vi "毕设原版.vi"() -> ()   [LabVIEW 2018]
uses:
  <vilib>/Utility/NIReport.llb/Report Type.ctl
  <vilib>/addons/control/pid/pid.llb/PID (DBL).vi
  <vilib>/Utility/NIReport.llb/Append Report Text (str wrap).vi
  <vilib>/express/express arith-compare/Formula/XNode/ExpressFormulaBlockNode.xnode
  <vilib>/Utility/NIReport.llb/NI_report.lvclass
  <vilib>/addons/control/pid/NI_PID_pid.lvlib
  <vilib>/Utility/NIReport.llb/NI_ReportGenerationCore.lvlib
  <vilib>/Utility/NIReport.llb/Excel/NI_Excel.lvclass
  <vilib>/Utility/NIReport.llb/Append Text Table to Report (wrap).vi
panel:
  out "波形图表":dbl(graph)
  out "过程变量和设定值 2":cluster{dbl, "SP：":dbl}(graph)
  in  "停止 3":bool
  out "实验要求":string="超    调    振    \n调    节    荡\n量    时    频\n不    间    率\n超    小    小\n过    于    于\n10   15    0.7\n%     s   rad/s"
  in  "密码修改":bool
  out "error out 6":errorcluster caption="error out"
  out "error out 5":errorcluster caption="error out"
  out "error out 4":errorcluster caption="error out"
  out "Values":string
  out "Command Text":string
  out "error out 2":errorcluster caption="错误输出"
  out "y":dbl[](array[numeric])
  out "time":dbl[](array[numeric])
  out "source":string
  out "Data":string[][](array[string])=[["10152949", "987654", "student"], ["10152950", "123456", "student"], ["10152951", "654321", "teacher"], ["10152952", "283411", "administrator"]]
  out "error out 3":errorcluster caption="error out"
  in  "report file path":path=path "F:/LabVIEW练习/毕设/实验成绩.xls"
  out "尝试次数":u32
  in  "text data":string[][](array[string])=[["1", "2"], ["3", "4"]]
  out "error out":errorcluster
  in  "超限累计":i32
  in  "文本方向":u16(ring) items=["None", "Stacked", "Clockwise", "Counterclockwise"]
  out "权限":enum16{"student", "teacher", "administrator"}(ring)=enum."administrator"
  out "数值 3":i32=191
  out "数值 2":dbl=44.692359011378294
  out "数组":dbl[](array[numeric])=[0.15946790534816901, 0.35556228083290553, 0.5907826417638008, 0.8494826417638008, 1.1081826417638008, 1.3668826417638007, 1.6255826417638006, 1.8842826417638006, 2.1429826417638007, 2.401682641763801, 2.660382641763801, 2.919082641763801, 3.1777826417638013, 3.4364826417638015, 3.6951826417638016, 3.9538826417638018, 4.2125826417638015, 4.471282641763802, 4.729982641763802, 4.988682641763802, 5.247382641763802, 5.506082641763802, 5.764782641763802, 6.0234826417638025, 6.282182641763803, 6.540882641763803, 6.799582641763803, 7.058282641763803, 7.316982641763803, 7.5756826417638035, 7.834382641763804, 8.093082641763804, 8.351782641763803, 8.610482641763802, 8.869182641763802, 9.1278826417638, 9.3865826417638, 9.6452826417638, 9.903982641763799, 10.162682641763798, 10.421382641763797, 10.680082641763796, 10.938782641763796, 11.197482641763795, 11.456182641763794, 11.714882641763793, 11.973582641763793, 12.232282641763792, 12.490982641763791, 12.74968264176379, 13.00838264176379, 13.267082641763789, 13.525782641763788, 13.784482641763788, 14.043182641763787, 14.301882641763786, 14.560582641763785, 14.819282641763785, 15.077982641763784, 15.336682641763783, 15.595382641763782, 15.854082641763782, 16.112782641763783, 16.371482641763784, 16.630182641763785, 16.888882641763786, 17.147582641763787, 17.406282641763788, 17.66498264176379, 17.92368264176379, 18.18238264176379, 18.441082641763792, 18.699782641763793, 18.958482641763794, 19.217182641763795, 19.475882641763796, 19.734582641763797, 19.9932826417638, 20.2519826417638, 20.5106826417638, 20.7693826417638, 21.028082641763802, 21.286782641763804, 21.545482641763805, 21.804182641763806, 22.062882641763807, 22.321582641763808, 22.58028264176381, 22.83898264176381, 23.09768264176381, 23.356382641763812, 23.615082641763813, 23.873782641763814, 24.132482641763815, 24.391182641763816, 24.649882641763817, 24.908582641763818, 25.16728264176382, 25.42598264176382, 25.68468264176382, 25.943382641763822, 26.202082641763823, 26.460782641763824, 26.719482641763825, 26.978182641763826, 27.236882641763827, 27.49558264176383, 27.75428264176383, 28.01298264176383, 28.27168264176383, 28.530382641763833, 28.789082641763834, 29.047782641763835, 29.306482641763836, 29.565182641763837, 29.823882641763838, 30.08258264176384, 30.34128264176384, 30.59998264176384, 30.858682641763842, 31.117382641763843, 31.376082641763844, 31.634782641763845, 31.893482641763846, 32.152182641763844, 32.41088264176384, 32.66958264176384, 32.928282641763836, 33.186982641763834, 33.44568264176383, 33.70438264176383, 33.963082641763826, 34.221782641763824, 34.48048264176382, 34.73918264176382, 34.997882641763816, 35.25658264176381, 35.51528264176381, 35.77372176165425, 36.031884459742486, 36.289771162313485, 36.54738216334767, 36.80471775760098, 37.061778239505244, 37.318522130243544, 37.57467358720941, 37.8299594264456, 38.084107940043786, 38.33686499688974, 38.587925999781845, 38.837015689907915, 39.08390098833731, 39.32828579607282, 39.56990831464298, 39.80852799499046, 40.04390159016064, 40.275777925533525, 40.503874950422215, 40.72793097876865, 40.94778181593828, 41.16322788169536, 41.3740472034328, 41.580023389427126, 41.78087973060037, 41.97645279482925, 42.166568681508785, 42.35103471778728, 42.52957941340393, 42.70208708634859, 42.86840732714809, 43.02827548540423, 43.18150954430742, 43.32806311134, 43.46781164646614, 43.600619222636375, 43.726357743660884, 43.84490694692867, 43.956154516980234, 44.05986646431542, 44.15606406402364, 44.24453639469577, 44.32519057948923, 44.39795443410196, 44.462764470554774, 44.51956602229976, 44.5684623722877, 44.60942425329443, 44.64227082069252, 44.666977641637374, 44.683534283119904, 44.69193920908696, 44.692359011378294, 44.68465028908381, 44.668999121914815, 44.64527563307593, 44.61352408042584, 44.57379545987751, 44.52614939302406, 44.47081710257968, 44.407867701626955, 44.3372216673248, 44.25897957356577, 44.17340367346343, 44.0804305099236, 43.98034675420013, 43.87326265304072, 43.75930728668722, 43.63846143518952, 43.511038790252734, 43.377022593732704, 43.23673818240778, 43.09033207622225, 42.93782851259838, 42.77956724262933, 42.615570642290564, 42.44618643585735, 42.271586813576505, 42.091838302223536, 41.90729733314443, 41.71802441898804, 41.52425881526584, 41.32633897695649, 41.12446160950261, 40.918741029655656, 40.70954089926177, 40.4969648106794, 40.281375841949064, 40.06298482798073, 39.84203160577297, 39.61875810290718, 39.39332769049512, 39.166094497507856, 38.937206459131936, 38.707011747084934, 38.47566953230472, 38.24346340376417, 38.01064870010497, 37.7774810808516, 37.54421607075162, 37.31114593136907, 37.07849129310784, 36.84650071747841, 36.615378575927984, 36.38537198581724, 36.156943040417275, 35.93015564000529, 35.70525048381508, 35.482464651506554, 35.26203247520919, 35.04418528714419, 34.82918977838842, 34.61728362150174, 34.40866418976721, 34.203545417677866, 34.002152710466156, 33.80468049370989, 33.611355630079316, 33.42235243373588, 33.237840660649525, 33.058071096130554, 32.88318656057269, 32.71334221077529, 32.548785239587595, 32.38970558748683, 32.23635039277429, 32.0887213027308, 31.94692772347299, 31.811109866020686, 31.681500382105583, 31.558141994624826, 31.441138071257893, 31.330710906159855, 31.226982177337977, 31.130051544807788, 31.03989192894575, 30.956574187060063, 30.880298416516695, 30.811016574667573, 30.748779172798816, 30.693770570174408, 30.64604383266606, 30.605500125335514, 30.57216235661245, 30.546191212341355, 30.52746301020953, 30.515979813151755, 30.511739148217686, 30.514730768837623, 30.525082405205367, 30.54262096493095, 30.567314262688704, 30.599121227790977, 30.63799326089107, 30.684022094229924, 30.737138109376353, 30.79712134083411, 30.864047204647928, 30.937674402846334, 31.01791864742922, 31.104680413124612, 31.197997533983642, 31.297601112667355, 31.403524770877823, 31.51548742435686, 31.633369889626856, 31.75717052786516, 31.886727545997974, 32.02188775690319, 32.16249207258547, 32.30824736260859, 32.45925547191968, 32.615179595589765, 32.77573670801291, 32.940882235017824, 33.110406544352976, 33.28411560358437, 33.46181107958789, 33.64318536552284, 33.82805847807178, 34.01632346763871, 34.20774500171118, 34.40210761886112, 34.59910568351407, 34.79863001296244, 35.00043309118822, 35.20421455937076, 35.409776861426906, 35.616895997678924, 35.82540967343328, 36.03500330478898, 36.245529997989294, 36.45673189274724, 36.66833177613277, 36.88016878368664, 37.09198479004521, 37.30354852280296, 37.514602306871495, 37.72494707482634, 37.93437652215988, 38.142624707699454, 38.349505294607624, 38.5547654289942, 38.758213276831206, 38.95961027411947, 39.15877000170116, 39.355468869927705, 39.54949168753746, 39.74066037677261, 39.92877582472998, 40.11361003289667, 40.29498171485171, 40.47268498177152, 40.64651067819616, 40.816326941874074, 40.98192711472907, 41.14317621204567, 41.29986838770229, 41.451821738844906, 41.5988799580375, 41.7409664432832, 41.87795719408764, 42.0097157520009, 42.13611165526278, 42.257020452567055, 42.372232010346224, 42.481617154649165, 42.585166458979025, 42.6826931531345, 42.774090098791774, 42.859376819902224, 42.938376129353465, 43.0110039302606, 43.0773083298165, 43.13700634690593, 43.19026686553209, 43.23706044447938, 43.27722730725126, 43.310855788692564, 43.33780207941015, 43.35817371768441, 43.37183675931807, 43.37878738416311, 43.379031648389216, 43.372714902851996, 43.35985733742113, 43.340486081998, 43.31463518904689, 43.28234558282003, 43.2436650014862, 43.198513698357374, 43.14695891512083, 43.08906997124019, 43.024922996561216, 42.95460080492671, 42.878324985411076, 42.79604942541201, 42.708016010792086, 42.61432063883826, 42.51494734919351, 42.41015434896103, 42.299927660461705, 42.184411727942404, 42.06386503485702, 41.938293151587985, 41.80785840805722, 41.672713132822174, 41.53312773424592, 41.389244209130915, 41.241117376020824, 41.08893540101152, 40.932975542979875, 40.77329393535387, 40.61018892311368, 40.44382249205406, 40.27428885036583, 40.10180013164225, 39.926634944570246, 39.74896521510243, 39.568986518363765, 39.38689637097467, 39.20289414894689, 39.017114489970886, 38.82984923352281, 38.641279065899965, 38.45160880070593, 38.2609929339156, 38.06966498568467, 37.87787826534298, 37.68577681806894]
  out "数值":i32=429
  in  "选项卡控件":T1(tab)=enum."实验二"
  in  "注册":T2
  in  "登录":T3
  in  "密码":string="283411"
  in  "字符串":string="10152952"
  in  "公告栏":string[](array[string])=["欢迎您试用本实验平台", "本次的实验内容有", "1xxxxxxxx", "2cccccccc", "3dddddd", "4xxxxxxxx", "5vvvvvvvv"]
  in  "确定":bool
  out "图片":picture caption="新图片"
  out "尝试次数":string
  in  "提交":bool
  out "可否提交":bool
  out "是否合格":T4
  out "动态性能指标":T5
  in  "开始":bool
  in  "停止":bool
  out "操作变量":dbl(graph)
  out "MV：":dbl(slide) scale=-100.0..100.0
  in  "SP：":dbl(slide) min=0.0 max=0.0 scale=0.0..120.0
  out "PV：":dbl(slide) scale=0.0..120.0
  in  "PID增益":T6={"比例增益(Kc)"=1.0, "积分时间（Ti，分）"=0.002, "微分时间（Td，分）"=0.002} {"微分时间（Td，分）" format="%.3f"; "积分时间（Ti，分）" format="%.3f"; "比例增益(Kc)" format="%.3f"}
  out "过程变量和设定值":cluster{dbl, "SP：":dbl}(graph)
  out "波形图":dbl[](graph)
  in  "开始2":bool
  in  "对象特性设置":cluster{"num":dbl[], "den":dbl[]}={"num"=[1.0], "den"=[0.02, 1.0]}
  in  "PID增益":cluster{"Kp":dbl, "Ki":dbl, "Kd":dbl}={"Kp"=1.5, "Ki"=0.35, "Kd"=1.0}
  in  "SP":dbl(slide) min=0.0 max=0.0 scale=0.0..120.0
  out "XY图":cluster{dbl[], dbl[]}(graph)
  in  "停止 2":bool
  out "超调量":dbl
  out "调节时间":dbl
  out "上升时间":dbl
  in  "姓名:":string="小明"
  in  "学号:":i32=10152949
  in  "确认提交":bool
  in  "File path of populated Word document":path=path "F:/LabVIEW练习/毕设/实验报告.doc"
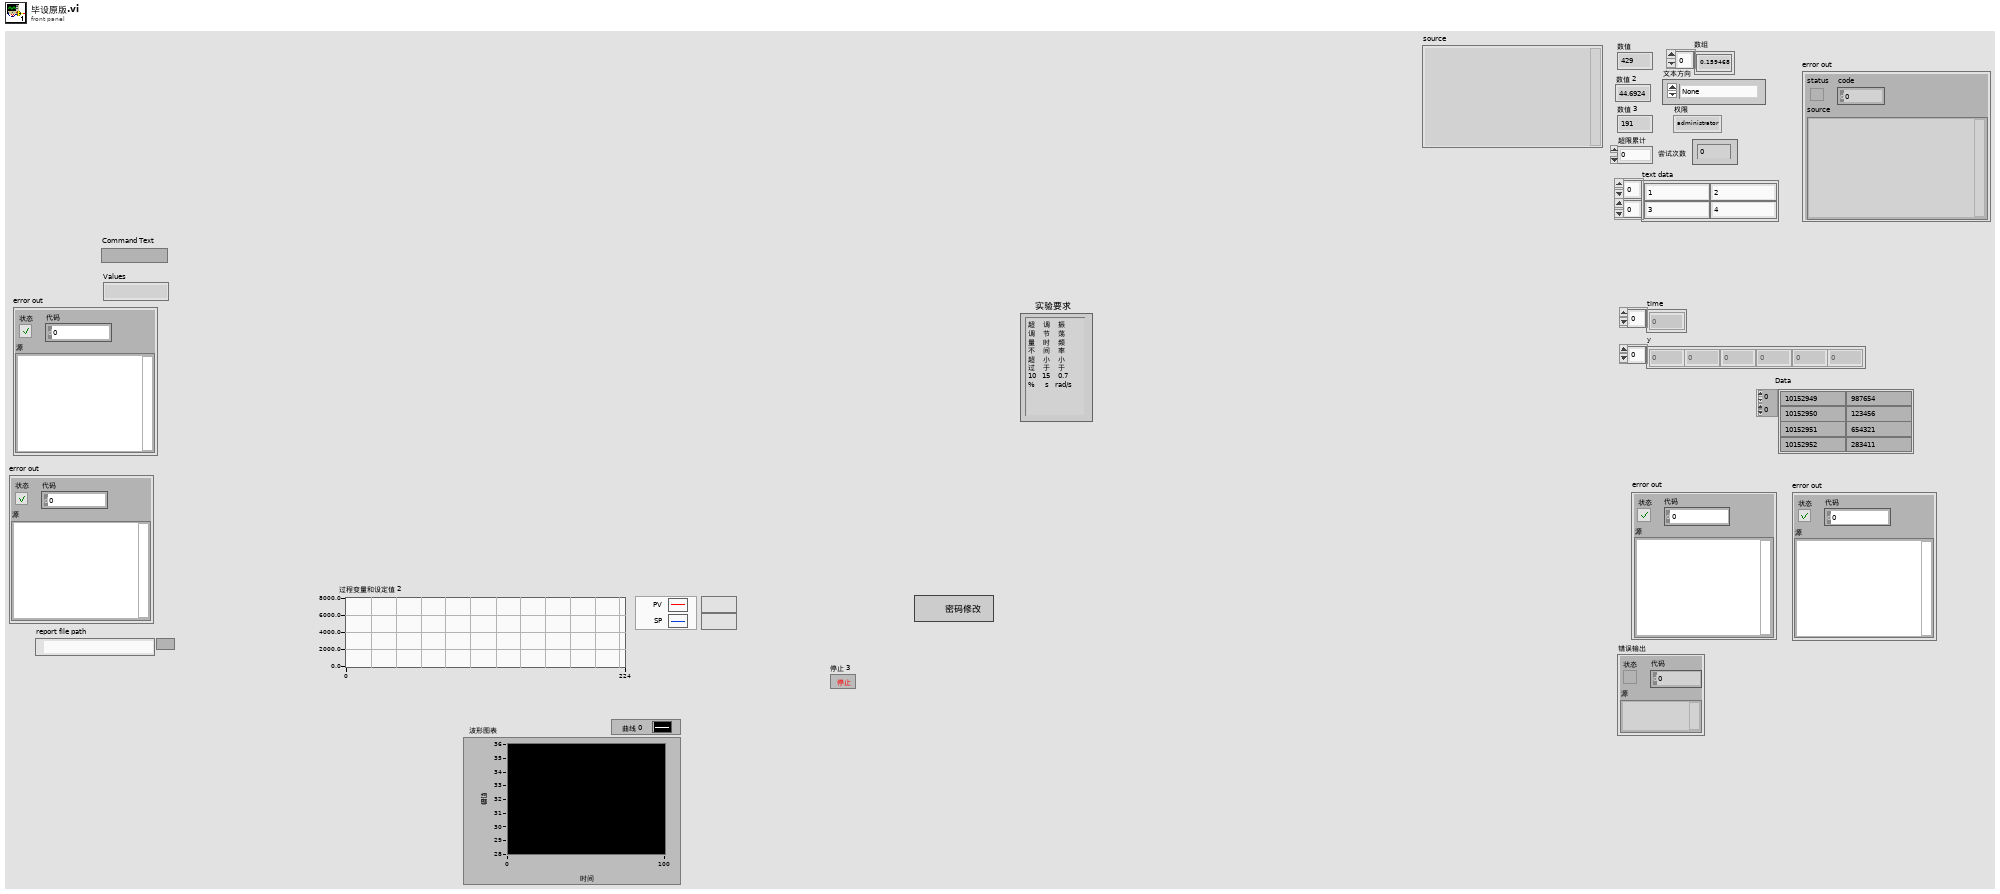
[diagram p1: front panel]
types:
  T1 = enum32{"登录", "公告", "实验一", "实验一历史曲线", "实验二", "提交页面"}
  T2 = typedef "注册.ctl" = bool
  T3 = typedef "登录.ctl" = bool
  T4 = cluster{"超调量":string, "振荡频率":string, "调节时间":string}
  T5 = cluster{"超调量":string, "振荡频率":string, "调节时间":string, " 峰值时间":string, "阻尼比 ":string}
  T6 = cluster{"比例增益(Kc)":dbl, "积分时间（Ti，分）":dbl, "微分时间（Td，分）":dbl}
  T7 = enum16{"User-specified Font", "Application Font", "System Font", "Dialog Font"}
  T8 = cluster{"Font Name:":string, "Size":i16, "Strikeout?":bool, "Italic?":bool, bool, "Outline?":bool, "Shadow?":bool, "Bold?":bool}
  T9 = enum8{"Enabled", "Disabled", "Disabled and Grayed Out"}
  T10 = cluster{"position (Excel)":cluster{"row":i32, "column":i32}, "name (Excel)":string, "bookmark (Word)":string}
  T11 = typedef "NI_ReportGenerationCore.lvlib/Report Type.ctl" = enum16{"HTML", "Word", "Excel"}
  T12 = cluster{"position (excel)":cluster{"row":i32, "column":i32}, "name (excel)":string, "bookmark (word)":string}
  T13 = cluster{cluster{"row":i32, i32}, "name (excel)":string, "bookmark (word)":string}
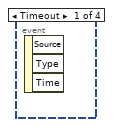
[diagram p3: hidden frame]
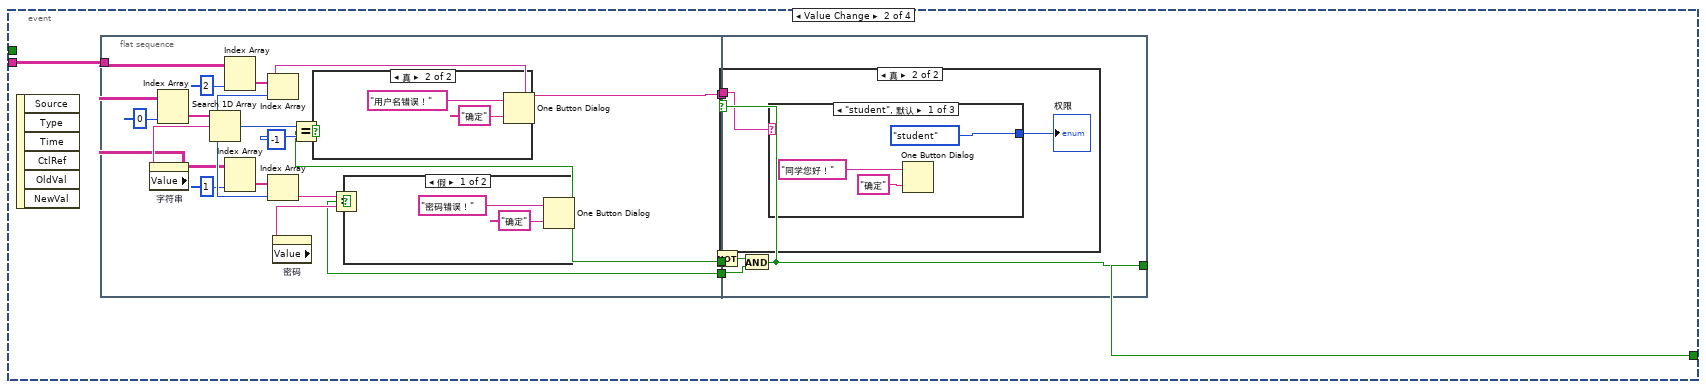
[diagram p4: hidden frame]
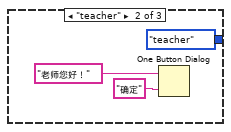
[diagram p8: hidden frame]
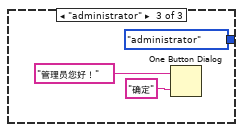
[diagram p9: hidden frame]
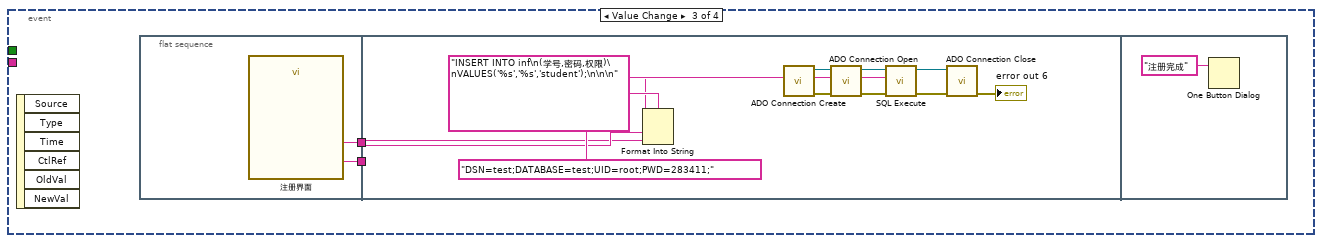
[diagram p10: hidden frame]
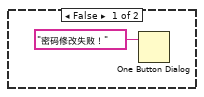
[diagram p11: hidden frame]
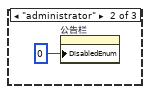
[diagram p12: hidden frame]
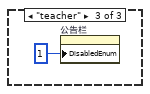
[diagram p13: hidden frame]
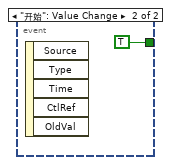
[diagram p14: hidden frame]
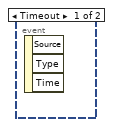
[diagram p16: hidden frame]
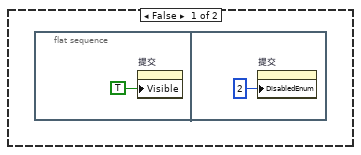
[diagram p19: hidden frame]
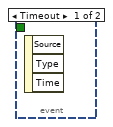
[diagram p20: hidden frame]
diagram:
  n1 = flat-sequence {
    frame #0 {
      n2 = flat-sequence {
        frame #0 {
          n3 = while {
            stop <- w22 stop-if-true
            n4 = property on="选项卡控件" class="TabCtl (严格)"() -> ("Pages"=w43:refnum<vi>[])  [unwired: 2 in, 2 out]
            n5 = property on="选项卡控件" class="TabCtl (严格)"() -> ("Pages"=w31:refnum<vi>[])  [unwired: 2 in, 2 out]
            n6 = property on="选项卡控件" class="TabCtl (严格)"() -> ("Pages"=w37:refnum<vi>[])  [unwired: 2 in, 2 out]
            n7 = property on="选项卡控件" class="TabCtl (严格)"() -> ("Pages"=w40:refnum<vi>[])  [unwired: 2 in, 2 out]
            n8 = property on="选项卡控件" class="TabCtl (严格)"() -> ("Pages"=w13:refnum<vi>[])  [unwired: 2 in, 2 out]
            n9 = property on="选项卡控件" class="TabCtl (严格)"() -> ("Pages"=w34:refnum<vi>[])  [unwired: 2 in, 2 out]
            n10 = Index Array(array=w31, index=T1."实验二" ("选项卡控件")) -> (element=w30:refnum<vi>)
            n11 = Index Array(array=w40, index=T1."实验一" ("选项卡控件")) -> (element=w41:refnum<vi>)
            n12 = Index Array(array=w13, index=T1."提交页面" ("选项卡控件")) -> (element=w15:refnum<vi>)
            n13 = Index Array(array=w43, index=T1."登录" ("选项卡控件")) -> (element=w42:refnum<vi>)
            n14 = Index Array(array=w37, index=T1."公告" ("选项卡控件")) -> (element=w36:refnum<vi>)
            n15 = Index Array(array=w34, index=T1."实验一历史曲线" ("选项卡控件")) -> (element=w35:refnum<vi>)
            n16 = property class="Page"(reference=w30, "PageVis"=FALSE ("选项卡可见")) -> ()  [unwired: 1 in, 2 out]
            n17 = property class="Page"(reference=w41, "PageVis"=FALSE) -> ()  [unwired: 1 in, 2 out]
            n18 = property class="Page"(reference=w15, "PageVis"=FALSE ("选项卡可见")) -> ()  [unwired: 1 in, 2 out]
            n19 = property class="Page"(reference=w42, "PageVis"=TRUE ("选项卡可见")) -> ()  [unwired: 1 in, 2 out]
            n20 = property class="Page"(reference=w36, "PageVis"=FALSE ("选项卡可见")) -> ()  [unwired: 1 in, 2 out]
            n21 = property class="Page"(reference=w35, "PageVis"=FALSE ("选项卡可见")) -> ()  [unwired: 1 in, 2 out]
            n22 = while {
              tunnel: [w49] -> w45
              stop <- w49 stop-if-true
              n23 = Compound Arithmetic op=OR ("复合运算")("登录", "注册", "密码修改") -> (w49:T3)
              n24 = Wait For Front Panel Activity(3:w49) -> ()  [unwired: 2 in, 1 out]
            }
            n25 = call <userlib>:"ADO Connection Create.vi"() -> ("error out"=w29:errorcluster, "ADODB._Connection Out"=w11:refnum<k7>)  [unwired: 10 in]
            n26 = call <userlib>:"ADO Connection Open.vi"("error in (no error)"=w29, "ConnectionString"="DSN=test;DATABASE=test;UID=root;PWD=283411;", "ADODB._Connection In"=w11) -> ("error out"=w28:errorcluster, "ADODB._Connection Out"=w10:refnum<k7>)  [unwired: 7 in]
            n27 = call <userlib>:"SQL Execute.vi"("error in (no error)"=w28, "Command Text"="SELECT * FROM inf;", "ADODB._Connection In"=w10) -> ("error out"=w27:errorcluster, "Data"=w23:string[][], "ADODB._Connection Out"=w12:refnum<k7>)  [unwired: 5 in, 1 out]
            "Data" <- w23
            n28 = event shown="[3] \"密码修改\": 值改变" {
              selector: _ -> [_ _ _ _]
              dyn-events: _ -> [_ _ _ _]
              timeout: _ -> [_ _ _ _]
              tunnel: w45 -> [_ _ _ _]
              tunnel: w23 -> [_ w50 _ w107]
              tunnel: [_ w51 _ _] -> w22
              event Timeout {
                n29 = event-data() -> ()  [unwired: 1 in, 3 out]
              }
              event Value Change {
                n30 = event-data() -> ()  [unwired: 1 in, 6 out]
                n31 = flat-sequence {
                  tunnel: w50 -> [w55]
                  tunnel: [w58] -> w54
                  tunnel: [w57] -> w53
                  tunnel: [w56] -> w52
                  tunnel: w54 -> [w75]
                  tunnel: w53 -> [w78]
                  tunnel: w52 -> [w76]
                  tunnel: [w74] -> w51
                  frame #0 {
                    n32 = property on="字符串" class="Str"() -> ("Value"=w64:string)  [unwired: 2 in, 2 out]
                    n33 = Index Array(array=w55, index (col)=0 ("禁用的索引 (列)")) -> (element=w63:string[])  [unwired: 1 in]
                    n34 = Search 1D Array(1D array=w63, element=w64) -> (index of element=w69:i32)  [unwired: 1 in]
                    n35 = Index Array(array=w55, index (col)=2 ("禁用的索引 (列)")) -> (element=w68:string[])  [unwired: 1 in]
                    n36 = Index Array(array=w55, index (col)=1 ("禁用的索引 (列)")) -> (element=w65:string[])  [unwired: 1 in]
                    n37 = Index Array(array=w68, index=w69) -> (element=w58:string)
                    n38 = Index Array(array=w65, index=w69) -> (element=w66:string)
                    n39 = property on="密码" class="Str"() -> ("Value"=w67:string)  [unwired: 2 in, 2 out]
                    n40 = Equal?(x=w69, y=-1) -> (x = y?=w56:bool)
                    n41 = case shown="真" w56 {
                      frame False {
                      }
                      frame True {
                        n42 = One Button Dialog(message="用户名错误！", button name ("OK")="确定" ("按钮名称（“确定”）")) -> ()  [unwired: 1 out]
                      }
                    }
                    n43 = Equal?(x=w66, y=w67) -> (x = y?=w57:bool)
                    n44 = case shown="假" w57 {
                      frame False {
                        n45 = One Button Dialog(message="密码错误！", button name ("OK")="确定" ("按钮名称（“确定”）")) -> ()  [unwired: 1 out]
                      }
                      frame True {
                      }
                    }
                  }
                  frame #1 {
                    n46 = Not(x=w76) -> (.not. x?=w77:bool)
                    n47 = And(x=w77, y=w78) -> (x .and. y?=w74:bool)
                    n48 = case shown="真" w74 {
                      tunnel: w75 -> [_ w79]
                      frame False {
                      }
                      frame True {
                        n49 = case shown="\"student\", 默认" w79 {
                          tunnel: [enum16{"student", "teacher", "administrator"}."student" ("枚举") enum16{"student", "teacher", "administrator"}."teacher" ("枚举") enum16{"student", "teacher", "administrator"}."administrator" ("枚举")] -> w80
                          frame "student", Default {
                            n50 = One Button Dialog(message="同学您好！", button name ("OK")="确定" ("按钮名称（“确定”）")) -> ()  [unwired: 1 out]
                          }
                          frame "teacher" {
                            n51 = One Button Dialog(message="老师您好！", button name ("OK")="确定" ("按钮名称（“确定”）")) -> ()  [unwired: 1 out]
                          }
                          frame "administrator" {
                            n52 = One Button Dialog(message="管理员您好！", button name ("OK")="确定" ("按钮名称（“确定”）")) -> ()  [unwired: 1 out]
                          }
                        }
                        "权限" <- w80
                      }
                    }
                  }
                }
              }
              event Value Change {
                n53 = event-data() -> ()  [unwired: 1 in, 6 out]
                n54 = flat-sequence {
                  tunnel: [w93] -> w91
                  tunnel: [w92] -> w90
                  tunnel: w91 -> [w99]
                  tunnel: w90 -> [w98]
                  frame #0 {
                    n55 = call "注册界面"() -> ("输入密码"=w92:string, "输入学/工号"=w93:string)  [unwired: 16 in, 2 out]
                  }
                  frame #1 {
                    n56 = Format Into String(format string="INSERT INTO inf\n(学号,密码,权限)\nVALUES('%s','%s','student');\n\n\n" ("Command Text"), w99, w98) -> (resulting string=w97:string)  [unwired: 2 in, 1 out]
                    n57 = call <userlib>:"ADO Connection Create.vi"() -> ("error out"=w104:errorcluster, "ADODB._Connection Out"=w103:refnum<k7>)  [unwired: 10 in]
                    n58 = call <userlib>:"ADO Connection Open.vi"("error in (no error)"=w104, "ConnectionString"="DSN=test;DATABASE=test;UID=root;PWD=283411;", "ADODB._Connection In"=w103) -> ("error out"=w105:errorcluster, "ADODB._Connection Out"=w102:refnum<k7>)  [unwired: 7 in]
                    n59 = call <userlib>:"SQL Execute.vi"("error in (no error)"=w105, "Command Text"=w97, "ADODB._Connection In"=w102) -> ("error out"=w94:errorcluster, "ADODB._Connection Out"=w95:refnum<k7>)  [unwired: 5 in, 2 out]
                    n60 = call <userlib>:"ADO Connection Close.vi"("error in (no error)"=w94, "ADODB._Connection In"=w95) -> ("error out"=→"error out 6":errorcluster)  [unwired: 8 in, 1 out]
                  }
                  frame #2 {
                    n61 = One Button Dialog(message="注册完成" ("消息")) -> ()  [unwired: 1 in, 1 out]
                  }
                }
              }
              event "密码修改": Value Change {
                n62 = event-data() -> ()  [unwired: 1 in, 6 out]
                n63 = flat-sequence {
                  tunnel: w107 -> [w116]
                  frame #0 {
                    n64 = Index Array(array=w116, index (col)=1 ("禁用的索引 (列)")) -> (element=w121:string[])  [unwired: 1 in]
                    n65 = Index Array(array=w116, index (col)=0 ("禁用的索引 (列)")) -> (element=w120:string[])  [unwired: 1 in]
                    n66 = call "密码更改"() -> ("再次输入新密码"=w109:string, "输入新密码"=w110:string, "输入原密码"=w108:string, "输入学/工号"=w111:string)  [unwired: 14 in, 2 out]
                    n67 = Equal?(x=w110, y=w109) -> (x = y?=w114:bool)
                    n68 = Search 1D Array(1D array=w120, element=w111) -> (index of element=w122:i32)  [unwired: 1 in]
                    n69 = Equal?(x=w122, y=-1) -> ()  [unwired: 1 out]
                    n70 = Index Array(array=w121, index=w122) -> (element=w115:string)
                    n71 = Equal?(x=w108, y=w115) -> (x = y?=w113:bool)
                    n72 = And(x=w114, y=w113) -> (x .and. y?=w112:bool)
                    n73 = case shown="真" w112 {
                      tunnel: w111 -> [_ w131]
                      tunnel: w110 -> [_ w130]
                      tunnel: w110 -> [_ w128]
                      frame False {
                        n74 = One Button Dialog(message="密码修改失败！" ("消息")) -> ()  [unwired: 1 in, 1 out]
                      }
                      frame True {
                        w126 = 2 items=["adLockUnspecified"=-1, "adLockReadOnly"=1, "adLockPessimistic"=2, "adLockOptimistic"=3, "adLockBatchOptimistic"=4] ("LockType")
                        w127 = 2 items=["adOpenUnspecified"=-1, "adOpenForwardOnly"=0, "adOpenKeyset"=1, "adOpenDynamic"=2, "adOpenStatic"=3] ("CursorType")
                        n75 = Concatenate Strings("学号=" ("字符串"), w131) -> (w134:string)
                        "Command Text" <- w134
                        n76 = One Button Dialog(message="密码修改成功！" ("消息")) -> ()  [unwired: 1 in, 1 out]
                        n77 = call <userlib>:"ADO Connection Create.vi"() -> ("error out"=w143:errorcluster, "ADODB._Connection Out"=w142:refnum<k7>)  [unwired: 10 in]
                        n78 = call <userlib>:"ADO Connection Open.vi"("error in (no error)"=w143, "ConnectionString"="DSN=test;DATABASE=test;UID=root;PWD=283411;", "ADODB._Connection In"=w142) -> ("error out"=→"error out 5":errorcluster, "ADODB._Connection Out"=w144:refnum<k7>)  [unwired: 7 in]
                        n79 = call <userlib>:"ADO Recordset Create.vi"() -> ("error out"=w140:errorcluster, "ADODB._Recordset Out"=w141:refnum<k7>)  [unwired: 10 in]
                        n80 = call <userlib>:"ADO Recordset Open.vi"("ADODB._Recordset In"=w141, "ADODB._Connection In"=w144, "CursorType"=w127, "LockType"=w126, "error in (no error)"=w140, "Command Text"="SELECT * FROM inf;") -> ("ADODB._Recordset Out"=w139:refnum<k7>, "error out"=w138:errorcluster)  [unwired: 12 in]
                        n81 = call <userlib>:"ADO Recordset self design.vi"("ADODB._Recordset In"=w139, "Fields"=1, "Values"=w128, "error in (no error)"=w138, "Command Text"=w134) -> ("ADODB._Recordset Out"=w137:refnum<k7>, "error out"=w136:errorcluster)  [unwired: 13 in]
                        n82 = call <userlib>:"ADO Recordset Close.vi"("ADODB._Recordset In"=w137, "error in (no error)"=w136) -> ("error out"=→"error out 4":errorcluster)  [unwired: 16 in, 1 out]
                        "Values" <- w130
                      }
                    }
                  }
                }
              }
            }
            n83 = call <userlib>:"ADO Connection Close.vi"("error in (no error)"=w27, "ADODB._Connection In"=w12) -> ("error out"=→"error out 3":errorcluster)  [unwired: 8 in, 1 out]
          }
        }
        frame #1 {
          n84 = property on="权限" class="Enum (严格)"() -> ("Value"=w148:enum16{"student", "teacher", "administrator"})  [unwired: 2 in, 2 out]
          n85 = property on="选项卡控件" class="TabCtl (严格)"() -> ("Pages"=w151:refnum<vi>[])  [unwired: 2 in, 2 out]
          n86 = property on="选项卡控件" class="TabCtl (严格)"() -> ("Pages"=w154:refnum<vi>[])  [unwired: 2 in, 2 out]
          n87 = case shown="\"student\", 默认" w148 {
            frame "student", Default {
              n88 = property on="公告栏" class="Arr (严格)"("DisabledEnum"=1) -> ()  [unwired: 2 in, 2 out]
            }
            frame "administrator" {
              n89 = property on="公告栏" class="Arr (严格)"("DisabledEnum"=0) -> ()  [unwired: 2 in, 2 out]
            }
            frame "teacher" {
              n90 = property on="公告栏" class="Arr (严格)"("DisabledEnum"=1) -> ()  [unwired: 2 in, 2 out]
            }
          }
          n91 = Index Array(array=w151, index=T1."登录" ("选项卡控件")) -> (element=w152:refnum<vi>)
          n92 = Index Array(array=w154, index=T1."公告" ("选项卡控件")) -> (element=w153:refnum<vi>)
          n93 = property class="Page"(reference=w152, "PageVis"=FALSE ("选项卡可见")) -> ()  [unwired: 1 in, 2 out]
          n94 = property class="Page"(reference=w153, "PageVis"=TRUE ("选项卡可见")) -> ()  [unwired: 1 in, 2 out]
        }
        frame #2 {
          n95 = for {
            N: 100 -> [_]
            tunnel: u32 0 ("Color In") -> [w191]
            tunnel: [w189] -> w160 mode=indexing
            i -> [w190]
            n96 = call <vilib>:"Hilite Color.vi"("Percentage(30)"=w190, "Color In"=w191) -> ("Hilite"=w189:u32)  [unwired: 1 out]
          }
          n97 = Reverse 1D Array(array=w160) -> (reversed array=w161:u32[])
          n98 = Build Array (concatenate) "创建数组"(w161, w160) -> (w159:u32[])
          n99 = Array Size(array=w159) -> (size(s)=w158:i32)
          n100 = Array Size(array="公告栏") -> (size(s)=w162:i32)
          n101 = while {
            tunnel: "公告栏" -> [w173]
            tunnel: w162 -> [w171]
            tunnel: w159 -> [w168]
            tunnel: w158 -> [w166]
            i -> [w172]
            stop <- w167 stop-if-true
            n102 = Quotient & Remainder(x=w172, y=w171) -> (x-y*floor(x/y)=w170:i32)  [unwired: 1 out]
            n103 = Index Array(array=w173, index=w170) -> (element=w169:string)
            n104 = while {
              tunnel: w169 -> [w187]
              tunnel: w168 -> [w184] mode=indexing
              tunnel: ["确定"] -> w167
              tunnel: w166 -> [w178]
              i -> [w175]
              stop <- w180 stop-if-true
              n105 = Add(x=1, y=w175) -> (x+y=w176:i32)
              n106 = Wait (ms)(milliseconds to wait=u32 15 ("等待时间（毫秒）")) -> ()  [unwired: 1 out]
              n107 = Equal?(x=w176, y=w178) -> (x = y?=w177:bool)
              n108 = Or(x=w177, y="确定") -> (x .or. y?=w180:bool)
              n109 = call <vilib>:"Draw Text at Point.vi"("text orientation"="文本方向", "[user-specified font]"=T8 {"Font Name:"="应用程序字体", "Size"=28, "Strikeout?"=FALSE, "Italic?"=FALSE, TRUE, "Outline?"=FALSE, "Shadow?"=FALSE, "Bold?"=FALSE}, "text color(black)"=w184, "desired font(Application)"=T7."User-specified Font", "text"=w187, "origin"=cluster{"x":i16, "y":i16} {"x"=50, "y"=20}) -> ("new picture"=→"图片":picture)  [unwired: 4 in, 1 out]
            }
          }
        }
        frame #3 {
          n110 = property on="选项卡控件" class="TabCtl (严格)"() -> ("Pages"=w197:refnum<vi>[])  [unwired: 2 in, 2 out]
          n111 = property on="选项卡控件" class="TabCtl (严格)"() -> ("Pages"=w206:refnum<vi>[])  [unwired: 2 in, 2 out]
          n112 = property on="选项卡控件" class="TabCtl (严格)"() -> ("Pages"=w194:refnum<vi>[])  [unwired: 2 in, 2 out]
          n113 = property on="选项卡控件" class="TabCtl (严格)"() -> ("Pages"=w212:refnum<vi>[])  [unwired: 2 in, 2 out]
          n114 = property on="选项卡控件" class="TabCtl (严格)"() -> ("Pages"=w215:refnum<vi>[])  [unwired: 2 in, 2 out]
          n115 = property on="提交" class="Bool (严格)"("Visible"=FALSE) -> ()  [unwired: 2 in, 2 out]
          n116 = property on="选项卡控件" class="TabCtl (严格)"() -> ("Pages"=w209:refnum<vi>[])  [unwired: 2 in, 2 out]
          n117 = Index Array(array=w197, index=T1."实验二" ("选项卡控件")) -> (element=w198:refnum<vi>)
          n118 = Index Array(array=w194, index=T1."提交页面" ("选项卡控件")) -> (element=w193:refnum<vi>)
          n119 = Index Array(array=w212, index=T1."实验一" ("选项卡控件")) -> (element=w213:refnum<vi>)
          n120 = Index Array(array=w206, index=T1."公告" ("选项卡控件")) -> (element=w205:refnum<vi>)
          n121 = Index Array(array=w209, index=T1."实验一历史曲线" ("选项卡控件")) -> (element=w208:refnum<vi>)
          n122 = Index Array(array=w215, index=T1."登录" ("选项卡控件")) -> (element=w216:refnum<vi>)
          n123 = property class="Page"(reference=w198, "PageVis"=TRUE ("选项卡可见")) -> ()  [unwired: 1 in, 2 out]
          n124 = property class="Page"(reference=w193, "PageVis"=FALSE ("选项卡可见")) -> ()  [unwired: 1 in, 2 out]
          n125 = property class="Page"(reference=w213, "PageVis"=TRUE ("选项卡可见")) -> ()  [unwired: 1 in, 2 out]
          n126 = property class="Page"(reference=w205, "PageVis"=FALSE ("选项卡可见")) -> ()  [unwired: 1 in, 2 out]
          n127 = property class="Page"(reference=w208, "PageVis"=TRUE ("选项卡可见")) -> ()  [unwired: 1 in, 2 out]
          n128 = property class="Page"(reference=w216, "PageVis"=FALSE ("选项卡可见")) -> ()  [unwired: 1 in, 2 out]
        }
      }
      n129 = while {
        tunnel: [w7] -> w2
        tunnel: [w6] -> w1
        stop <- "停止 3" stop-if-true
        w6 = 30.0 ("Kp")
        n130 = Wait (ms)(milliseconds to wait=u32 100 ("毫秒计时值")) -> ()  [unwired: 1 out]
        n131 = shared-variable ".\\OPC变量.lvlib\\y2"() -> (w7:dbl)  [unwired: 1 in, 1 out]
        "波形图表" <- w7
        n132 = shared-variable "我的电脑\\OPC变量.lvlib\\Kp"(w6) -> ()  [unwired: 1 in, 1 out]
      }
      n133 = disable-structure shown="禁用" {
        disable-tunnel: w2 -> [w4 _]
        disable-tunnel: w1 -> [w3 _]
        frame Disabled {
          n134 = Bundle("Double"=w4, "Kp"=w3) -> (→"过程变量和设定值 2":cluster{"Double":dbl, "Kp":dbl})  [unwired: 1 in]
        }
        frame Enabled {
        }
      }
    }
    frame #1 {
      n135 = while {
        stop <- w217 stop-if-true
        n136 = flat-sequence {
          tunnel: [w279] -> w217
          frame #0 {
            n137 = while {
              stop <- w219 stop-if-true
              n138 = event shown="[0] 超时" {
                selector: _ -> [_ _]
                dyn-events: _ -> [_ _]
                timeout: 10 -> [_ _]
                tunnel: [FALSE TRUE] -> w219
                event Timeout {
                  n139 = event-data() -> ()  [unwired: 1 in, 3 out]
                }
                event "开始": Value Change {
                  n140 = event-data() -> ()  [unwired: 1 in, 5 out]
                }
              }
              n141 = case shown="真" "开始2" {
                frame False {
                }
                frame True {
                  n142 = while {
                    stop <- "停止 2" stop-if-true
                    n143 = Unbundle By Name("对象特性设置") -> ("num"=w227:dbl[], "den"=w226:dbl[])
                    n144 = Unbundle By Name("PID增益") -> ("Kp"=w231:dbl, "Ki"=w230:dbl, "Kd"=w229:dbl)
                    n145 = script code="ts=0.005;  %采样时间=0.05s\nsys=tf(num,den);   \ndsys=c2d(sys,ts,'z');      %离散化\n[num,den]=tfdata(dsys,'v');\ne_1=0;      %前一时刻的偏差      \nEe=0;       %累积偏差\nu_1=0.0;    %前一时刻的控制量\ny_1=0;       %前一时刻的输出\nu=zeros(1,100);\ntime=zeros(1,100);\nfor k=1:1:100\n    time(k)=k*ts;   %时间参数\n    r(k)=sp;      %给定量\n    y(k)=-1*den(2)*y_1+num(2)*u_1+num(1)*u(k);\n    e(k)=r(k)-y(k);   %偏差\n    u(k)=Kp*e(k)+Ki*Ee+Kd*(e(k)-e_1);   \n    Ee=Ee+e(k);    \n    u_1=u(k);    \n    y_1=y(k);    \n    e_1=e(k);\nend\nn=length(time);\n[ymax,ind]=max(y);\nyss=y(n);\ntp=time(ind);\nmp=100*(ymax-yss)/yss;\ny1=1.05*yss;\ny2=0.95*yss;\nk=n;\nwhile k>0\nk=k-1;\nif y(k)>=y1|y(k)<=y2;\nm=k;\nx=y(k);\nts=time(m);\nbreak;\nend\nend\nfor k=1:n\nif y(k)<=0.9*yss&y(k+1)>=0.9*yss\ntr=time(k);\nbreak\nend\nend"("Kp"=w231, "Ki"=w230, "Kd"=w229, "sp"="SP", "num"=w227, "den"=w226) -> ("time"=w236:dbl[], "y"=w235:dbl[], "mp"=→"超调量":dbl, "ts"=→"调节时间":dbl, "tr"=→"上升时间":dbl)  [unwired: 1 in, 1 out]
                    "time" <- w236
                    "y" <- w235
                    n146 = Bundle(w236, w235) -> (→"XY图":cluster{dbl[], dbl[]})  [unwired: 1 in]
                  }
                }
              }
            }
            n147 = flat-sequence {
              frame #0 {
                n148 = property on="开始" class="Bool (严格)"("DisabledEnum"=T9."Enabled" ("禁用")) -> ()  [unwired: 2 in, 2 out]
              }
              frame #1 {
                n149 = event shown="[1] \"开始\": 值改变" {
                  selector: _ -> [_ _]
                  dyn-events: _ -> [_ _]
                  timeout: _ -> [_ _]
                  event Timeout {
                    n150 = event-data() -> ()  [unwired: 1 in, 3 out]
                  }
                  event "开始": Value Change {
                    n151 = event-data() -> ()  [unwired: 1 in, 6 out]
                    n152 = property on="尝试次数" class="DigNum (严格)"() -> ("Value"=w241:u32)  [unwired: 2 in, 2 out]
                    n153 = local write "超限累计"(-1) -> ()
                    n154 = Add(x=w241, y=u32 1) -> (x+y=→"尝试次数":u32)
                    n155 = property on="开始" class="Bool (严格)"("DisabledEnum"=T9."Disabled and Grayed Out" ("禁用")) -> ()  [unwired: 2 in, 2 out]
                  }
                }
              }
            }
          }
          frame #1 {
            n156 = while {
              shift-right: [w261] -> _
              shift-left: 0 -> [w254]
              tunnel: [w261] -> w245 mode=indexing
              stop <- "停止" stop-if-true
              w256 = u32 6618880  # 正常
              w255 = u32 16711680  # 高压
              w257 = 100.0  # 高压
              n157 = Wait (ms)(milliseconds to wait=50) -> ()  [unwired: 1 out]
              n158 = Greater?(x=w254, y=w257) -> (0:w259:bool)
              n159 = In Range and Coerce "判定范围并强制转换"(upper limit=w257, x=w254, lower limit=0.0 ("下限")) -> (In Range?=w260:bool)  [unwired: 1 out]
              n160 = Bundle(w254, "SP："="SP：") -> (→"过程变量和设定值":cluster{dbl, "SP：":dbl})  [unwired: 1 in]
              n161 = call-poly <vilib>:"PID.vi"("PID gains"="PID增益", "process variable"=w254, "setpoint"="SP：") -> ("output"=w264:dbl)  [unwired: 7 in, 1 out]
              "MV：" <- w264
              "操作变量" <- w264
              n162 = Select "选择"(t=w255, s=w259, f=w256) -> (s? t:f=w253:u32)
              n163 = Multiply(x=w264, y=0.002587) -> (x*y=w269:dbl)
              n164 = Quotient & Remainder(x="超限累计", y=50) -> (x-y*floor(x/y)=w249:i32)  [unwired: 1 out]
              n165 = property on="PV：" class="Slide (严格)"("Fill Color"=w253) -> ()  [unwired: 2 in, 2 out]
              n166 = Not(x=w260) -> (.not. x?=w252:bool)
              n167 = Equal?(x=w249, y=0) -> (x = y?=w247:bool)
              n168 = case shown="真" w252 {
                frame False {
                }
                frame True {
                  n169 = local read "超限累计"() -> (w274:i32)
                  n170 = Add(x=w274, y=1) -> (x+y=w272:i32)
                  n171 = local write "超限累计"(w272) -> ()
                }
              }
              n172 = And(x=w252, y=w247) -> (x .and. y?=w246:bool)
              n173 = Multiply(x=w254, y=1.0) -> (x*y=w268:dbl)
              n174 = Add(x=w269, y=w268) -> (x+y=w261:dbl)
              n175 = case shown="真" w246 {
                frame False {
                }
                frame True {
                  n176 = One Button Dialog "单按钮对话框"(message="温度已经高于100，请尽快降低或停止！") -> ()  [unwired: 1 in, 1 out]
                }
              }
              "PV：" <- w254
            }
            "数组" <- w245
          }
          frame #2 {
            n177 = property on="尝试次数" class="DigNum (严格)"() -> ("Value"=w278:u32)  [unwired: 2 in, 2 out]
            n178 = property on="数组" class="Arr (严格)"() -> ("Value"=w276:dbl[])  [unwired: 2 in, 2 out]
            "波形图" <- w276
            n179 = Number To Decimal String(number=w278) -> (decimal integer string=→"尝试次数":string)  [unwired: 1 in]
            n180 = Array Size(array=w276) -> (size(s)=w321:i32)
            "数值" <- w321
            n181 = Array Max & Min(array=w276) -> (max value=w320:dbl, max index (indices)=w314:i32)  [unwired: 2 out]
            "数值 2" <- w320
            "数值 3" <- w314
            n182 = Subtract(x=w321, y=1) -> (x-y=w322:i32)
            n183 = Index Array(array=w276, index=w322) -> (element=w324:dbl)
            n184 = Subtract(x=w320, y=w324) -> (x-y=w323:dbl)
            n185 = Divide(x=w323, y=w324) -> (x/y=w309:dbl)
            n186 = xnode "公式"("X1"=w309) -> ("结果"=w303:dbl)  [unwired: 1 in, 1 out]
            n187 = Multiply(x=w314, y=0.05) -> (x*y=w307:dbl)
            n188 = xnode "公式 2"("X1"=w307, "X2"=w303) -> ("结果"=w288:dbl)  [unwired: 1 in, 1 out]
            n189 = xnode "公式 3"("X1"=w303, "X2"=w288) -> ("结果"=w291:dbl)  [unwired: 1 in, 1 out]
            n190 = Multiply(x=w309, y=100.0) -> (x*y=w293:dbl)
            n191 = Number To Fractional String(number=w293, precision (6)=2) -> (F-format string=w316:string)  [unwired: 2 in]
            n192 = Number To Fractional String(number=w288, precision (6)=2) -> (F-format string=w304:string)  [unwired: 2 in]
            n193 = Number To Fractional String(number=w291, precision (6)=2) -> (F-format string=w302:string)  [unwired: 2 in]
            n194 = Number To Fractional String(number=w307, precision (6)=2) -> (F-format string=w312:string)  [unwired: 2 in]
            n195 = Less Or Equal?(x=w293, y=10.0) -> (x <= y?=w283:bool)
            n196 = Less?(x=w291, y=15.0) -> (x < y?=w281:bool)
            n197 = Less?(x=w288, y=0.7) -> (x < y?=w282:bool)
            n198 = case shown="真" w283 {
              tunnel: ["不合格" "合格"] -> w287
              frame False {
              }
              frame True {
              }
            }
            n199 = case shown="真" w282 {
              tunnel: ["不合格" "合格"] -> w286
              frame False {
              }
              frame True {
              }
            }
            n200 = case shown="假" w281 {
              tunnel: ["不合格" "合格"] -> w285
              frame False {
              }
              frame True {
              }
            }
            n201 = Compound Arithmetic op=AND ("复合运算")(w283, w282, w281) -> (w280:bool)
            "可否提交" <- w280
            n202 = Concatenate Strings(w302, " s") -> (w297:string)
            n203 = Concatenate Strings(w312, " s") -> (w294:string)
            n204 = Concatenate Strings(w316, " %") -> (w299:string)
            n205 = Concatenate Strings(w304, " rad/s") -> (w296:string)
            n206 = Number To Fractional String(number=w303, precision (6)=2) -> (F-format string=w295:string)  [unwired: 2 in]
            n207 = Bundle(w299, w296, w297, w294, w295) -> (→"动态性能指标":cluster{string, string, string, string, string})  [unwired: 1 in]
            n208 = case shown="真" w280 {
              selector: w280 -> [_ w328]
              tunnel: [_ w327] -> w279
              frame False {
                n209 = flat-sequence {
                  frame #0 {
                    n210 = property on="提交" class="Bool (严格)"("Visible"=TRUE) -> ()  [unwired: 2 in, 2 out]
                  }
                  frame #1 {
                    n211 = property on="提交" class="Bool (严格)"("DisabledEnum"=2) -> ()  [unwired: 2 in, 2 out]
                  }
                }
              }
              frame True {
                n212 = flat-sequence {
                  tunnel: w328 -> [w329]
                  tunnel: [w331] -> w327
                  frame #0 {
                    n213 = property on="提交" class="Bool (严格)"("Visible"=w329) -> ()  [unwired: 2 in, 2 out]
                  }
                  frame #1 {
                    n214 = property on="提交" class="Bool (严格)"("DisabledEnum"=0) -> ()  [unwired: 2 in, 2 out]
                  }
                  frame #2 {
                    n215 = while {
                      tunnel: ["提交"] -> w332
                      stop <- "提交" stop-if-true
                      n216 = Wait For Front Panel Activity(3:"提交") -> ()  [unwired: 2 in, 1 out]
                    }
                    n217 = event shown="[1] \"提交\": 值改变" {
                      selector: _ -> [_ _]
                      dyn-events: _ -> [_ _]
                      timeout: _ -> [_ _]
                      tunnel: w332 -> [_ _]
                      tunnel: [_ TRUE] -> w331
                      event Timeout {
                        n218 = event-data() -> ()  [unwired: 1 in, 3 out]
                      }
                      event "提交": Value Change {
                        n219 = event-data() -> ()  [unwired: 1 in, 4 out]
                      }
                    }
                  }
                }
              }
            }
            n220 = Bundle(w287, w286, w285) -> (→"是否合格":cluster{string, string, string})  [unwired: 1 in]
          }
        }
      }
    }
    frame #2 {
      n221 = disable-structure shown="禁用" {
        frame Disabled {
          n222 = call-poly <vilib>:"Append Table to Report.vi"("MS Office parameters"=T10 {"position (Excel)"={"row"=0, "column"=0}, "name (Excel)"="", "bookmark (Word)"="data"} ("MS Office parameters 5"), "text data"="text data") -> ()  [unwired: 10 in, 4 out]
        }
        frame Enabled {
        }
      }
      n223 = flat-sequence {
        frame #0 {
          n224 = property on="选项卡控件" class="TabCtl (严格)"() -> ("Pages"=w371:refnum<vi>[])  [unwired: 2 in, 2 out]
          n225 = property on="选项卡控件" class="TabCtl (严格)"() -> ("Pages"=w382:refnum<vi>[])  [unwired: 2 in, 2 out]
          n226 = property on="选项卡控件" class="TabCtl (严格)"() -> ("Pages"=w386:refnum<vi>[])  [unwired: 2 in, 2 out]
          n227 = property on="选项卡控件" class="TabCtl (严格)"() -> ("Pages"=w385:refnum<vi>[])  [unwired: 2 in, 2 out]
          n228 = property on="选项卡控件" class="TabCtl (严格)"("Value"=T1."提交页面" ("选项卡控件")) -> ()  [unwired: 2 in, 2 out]
          n229 = Index Array(array=w371, index=T1."实验二" ("选项卡控件")) -> (element=w372:refnum<vi>)
          n230 = Index Array(array=w382, index=T1."实验一" ("选项卡控件")) -> (element=w383:refnum<vi>)
          n231 = Index Array(array=w386, index=T1."提交页面" ("选项卡控件")) -> (element=w387:refnum<vi>)
          n232 = Index Array(array=w385, index=T1."实验一历史曲线" ("选项卡控件")) -> (element=w384:refnum<vi>)
          n233 = property class="Page"(reference=w372, "PageVis"=FALSE ("选项卡可见")) -> ()  [unwired: 1 in, 2 out]
          n234 = property class="Page"(reference=w383, "PageVis"=FALSE ("选项卡可见")) -> ()  [unwired: 1 in, 2 out]
          n235 = property class="Page"(reference=w387, "PageVis"=TRUE ("选项卡可见")) -> ()  [unwired: 1 in, 2 out]
          n236 = property class="Page"(reference=w384, "PageVis"=FALSE ("选项卡可见")) -> ()  [unwired: 1 in, 2 out]
        }
        frame #1 {
          n237 = event shown="[1] \"确认提交\": 值改变" {
            selector: _ -> [_ _]
            dyn-events: _ -> [_ _]
            timeout: _ -> [_ _]
            tunnel: "确认提交" -> [_ _]
            event Timeout {
              n238 = event-data() -> ()  [unwired: 1 in, 3 out]
            }
            event "确认提交": Value Change {
              n239 = event-data() -> ()  [unwired: 1 in, 5 out]
            }
          }
        }
        frame #2 {
          n240 = call <vilib>:"Create Report.vi"("report type"=Report_Type."Excel", "template (empty)"=path "F:/LabVIEW练习/毕设/实验成绩.xls") -> ("report out"=w421:refnum<class "NI_report.lvclass">, "error out"=w420:errorcluster)  [unwired: 12 in]
          n241 = call <vilib>:"Create Report.vi"("report type"=Report_Type."Word", "template (empty)"=path "F:/LabVIEW练习/毕设/实验报告模板.doc") -> ("report out"=w451:refnum<class "NI_report.lvclass">, "error out"=w452:errorcluster)  [unwired: 12 in]
          n242 = call <vilib>:"Excel Get Last Row.vi"("report in"=w421, "error in (no error)"=w420) -> ("report out"=w418:refnum<class "NI_report.lvclass">, "MS Office parameters out"=w407:T12, "error out"=w419:errorcluster)  [unwired: 11 in]
          n243 = Get Date/Time String() -> (date string=w463:string, time string=w464:string)  [unwired: 3 in]
          n244 = Unbundle By Name(w407) -> ("position (excel)"=w408:cluster{"row":i32, "column":i32})
          n245 = call-poly <vilib>:"Append Report Text.vi"("report in"=w451, "MS Office parameters"=T12 {"position (excel)"={"row"=0, "column"=0}, "name (excel)"="", "bookmark (word)"="date"}, "text"=w463, "error in (no error)"=w452) -> ("report out"=w459:refnum<class "NI_report.lvclass">, "error out"=w460:errorcluster)  [unwired: 8 in, 2 out]
          n246 = Unbundle By Name(w408) -> ("row"=w397:i32)
          n247 = call-poly <vilib>:"Append Report Text.vi"("report in"=w459, "MS Office parameters"=T12 {"position (excel)"={"row"=0, "column"=0}, "name (excel)"="", "bookmark (word)"="time"} ("MS Office parameters 2"), "text"=w464, "error in (no error)"=w460) -> ("report out"=w465:refnum<class "NI_report.lvclass">, "error out"=w466:errorcluster)  [unwired: 8 in, 2 out]
          n248 = Bundle("row"=w397, 0) -> (w405:cluster{"row":i32, i32})  [unwired: 1 in]
          n249 = Number To Decimal String(number="学号:") -> (decimal integer string=w417:string)  [unwired: 1 in]
          n250 = Bundle("row"=w397, 1) -> (w399:cluster{"row":i32, i32})  [unwired: 1 in]
          n251 = Bundle(w405, "name (excel)"="", "bookmark (word)"="") -> (w402:T13)  [unwired: 1 in]
          n252 = call-poly <vilib>:"Append Report Text.vi"("report in"=w418, "MS Office parameters"=w402, "text"=w417, "error in (no error)"=w419) -> ("report out"=w413:refnum<class "NI_report.lvclass">, "error out"=w412:errorcluster)  [unwired: 8 in, 2 out]
          n253 = call-poly <vilib>:"Append Report Text.vi"("report in"=w465, "MS Office parameters"=T12 {"position (excel)"={"row"=0, "column"=0}, "name (excel)"="", "bookmark (word)"="姓名"} ("MS Office parameters 3"), "text"="姓名:", "error in (no error)"=w466) -> ("report out"=w467:refnum<class "NI_report.lvclass">, "error out"=w468:errorcluster)  [unwired: 8 in, 2 out]
          n254 = Bundle(w399, "name (excel)"="", "bookmark (word)"="") -> (w396:T13)  [unwired: 1 in]
          n255 = property on="动态性能指标" class="Clust (严格)"() -> ("Value"=w445:T5)  [unwired: 2 in, 2 out]
          n256 = call-poly <vilib>:"Append Report Text.vi"("report in"=w413, "MS Office parameters"=w396, "text"="姓名:", "error in (no error)"=w412) -> ("report out"=w410:refnum<class "NI_report.lvclass">, "error out"=w409:errorcluster)  [unwired: 8 in, 2 out]
          n257 = call-dynamic "Save Report to File.vi"("report in"=w410, "report file path"="report file path", "error in (no error)"=w409) -> ("report out"=w416:refnum<class "NI_report.lvclass">, "error out"=w415:errorcluster)  [unwired: 11 in]
          n258 = Unbundle(w445) -> ("超调量"=w430:string, "振荡频率"=w431:string, "调节时间"=w429:string, "峰值时间"=w428:string, "阻尼比"=w427:string)
          n259 = call-poly <vilib>:"Append Report Text.vi"("report in"=w467, "MS Office parameters"=T12 {"position (excel)"={"row"=0, "column"=0}, "name (excel)"="", "bookmark (word)"="学号"} ("MS Office parameters 4"), "text"=w417, "error in (no error)"=w468) -> ("report out"=w448:refnum<class "NI_report.lvclass">, "error out"=w447:errorcluster)  [unwired: 8 in, 2 out]
          n260 = call-dynamic "Dispose Report.vi"("report in"=w416, "error in (no error)"=w415) -> ("error out"=→"error out 2":errorcluster)  [unwired: 13 in]
          n261 = call-poly <vilib>:"Append Report Text.vi"("report in"=w448, "MS Office parameters"=T12 {"position (excel)"={"row"=0, "column"=0}, "name (excel)"="", "bookmark (word)"="超调量"}, "text"=w430, "error in (no error)"=w447) -> ("report out"=w443:refnum<class "NI_report.lvclass">, "error out"=w442:errorcluster)  [unwired: 8 in, 2 out]
          n262 = call-poly <vilib>:"Append Report Text.vi"("report in"=w443, "MS Office parameters"=T12 {"position (excel)"={"row"=0, "column"=0}, "name (excel)"="", "bookmark (word)"="振荡频率"}, "text"=w431, "error in (no error)"=w442) -> ("report out"=w437:refnum<class "NI_report.lvclass">, "error out"=w436:errorcluster)  [unwired: 8 in, 2 out]
          n263 = call-poly <vilib>:"Append Report Text.vi"("report in"=w437, "MS Office parameters"=T12 {"position (excel)"={"row"=0, "column"=0}, "name (excel)"="", "bookmark (word)"="调节时间"}, "text"=w429, "error in (no error)"=w436) -> ("report out"=w435:refnum<class "NI_report.lvclass">, "error out"=w434:errorcluster)  [unwired: 8 in, 2 out]
          n264 = call-poly <vilib>:"Append Report Text.vi"("report in"=w435, "MS Office parameters"=T12 {"position (excel)"={"row"=0, "column"=0}, "name (excel)"="", "bookmark (word)"="峰值时间"}, "text"=w428, "error in (no error)"=w434) -> ("report out"=w433:refnum<class "NI_report.lvclass">, "error out"=w432:errorcluster)  [unwired: 8 in, 2 out]
          n265 = call-poly <vilib>:"Append Report Text.vi"("report in"=w433, "MS Office parameters"=T12 {"position (excel)"={"row"=0, "column"=0}, "name (excel)"="", "bookmark (word)"="阻尼比"}, "text"=w427, "error in (no error)"=w432) -> ("report out"=w394:refnum<class "NI_report.lvclass">, "error out"=w392:errorcluster)  [unwired: 8 in, 2 out]
          n266 = control-ref of="波形图"() -> (w390:refnum<vi>)
          n267 = call-dynamic "Append Control Image to Report.vi"("report in"=w394, "ctrl reference"=w390, "error in (no error)"=w392, "MS Office parameters"=T10 {"position (Excel)"={"row"=0, "column"=0}, "name (Excel)"="", "bookmark (Word)"="实验图像"}) -> ("report out"=w393:refnum<class "NI_report.lvclass">, "error out"=w391:errorcluster)  [unwired: 8 in, 2 out]
          n268 = property on="尝试次数" class="Str"() -> ("Value"=w426:string)  [unwired: 2 in, 2 out]
          n269 = call-poly <vilib>:"Append Report Text.vi"("report in"=w393, "MS Office parameters"=T12 {"position (excel)"={"row"=0, "column"=0}, "name (excel)"="", "bookmark (word)"="尝试次数"}, "text"=w426, "error in (no error)"=w391) -> ("report out"=w425:refnum<class "NI_report.lvclass">, "error out"=w424:errorcluster)  [unwired: 8 in, 2 out]
          n270 = call-dynamic "Save Report to File.vi"("report in"=w425, "report file path"="File path of populated Word document", "error in (no error)"=w424) -> ("report out"=w461:refnum<class "NI_report.lvclass">, "error out"=w462:errorcluster)  [unwired: 11 in]
          n271 = call-dynamic "Dispose Report.vi"("report in"=w461, "error in (no error)"=w462) -> ("error out"=→"error out":errorcluster)  [unwired: 13 in]
        }
      }
    }
  }
